vi "Drive Reef Align Alternate_wrapper.vi"() -> ()   [LabVIEW 2023]
uses:
  <vilib>/Rock Robotics/WPI/Framework/Command Status Info.ctl
  <vilib>/Rock Robotics/WPI/Framework/Completion Status.ctl
  <vilib>/Rock Robotics/WPI/Framework/Completion Notifier.ctl
  swerve/Type Definitions/Data/Robot Velocities.ctl
  Implementation/Drive Operations.ctl
panel:
  in  "Operation":T1
  out "Command Info Out":T2
  in  "Description":string
  in  "Auto Data":T6
  in  "Robot Velocities":T5
  in  "Command Info In":T2
  in  "Left side":bool
  in  "Angle Align":bool
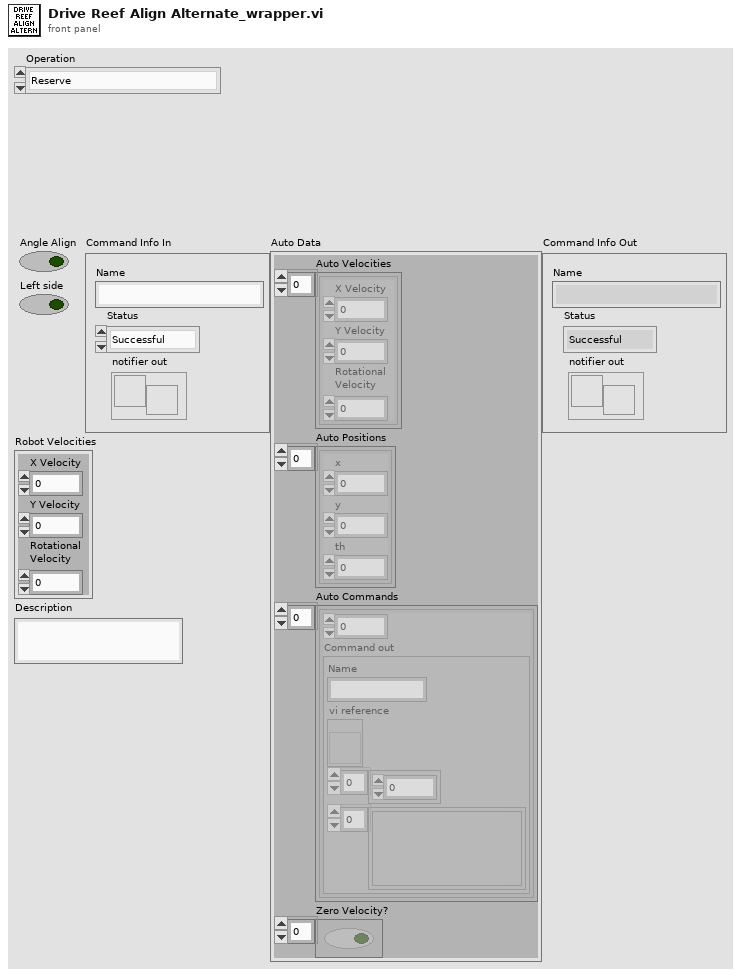
[diagram p1: front panel]
types:
  T1 = typedef "Drive Operations.ctl" = enum16{"Reserve", "Read Current", "Immediate", "Calibrate", "Reef Align", "Auto"}
  T2 = typedef "Command Status Info.ctl" = cluster{"Name":string, "Status":T3, "notifier out":T4}
  T3 = typedef "Completion Status.ctl" = enum16{"Successful", "Aborted", "Incomplete"}
  T4 = typedef "Completion Notifier.ctl" = refnum<notifier>
  T5 = typedef "Robot Velocities.ctl" = cluster{"X Velocity":dbl, "Y Velocity":dbl, "Rotational \nVelocity":dbl}
  T6 = cluster{"Auto Velocities":T5[], "Auto Positions":cluster{"x":dbl, "y":dbl, "th":dbl}[], "Auto Commands":cluster{dbl, "Command out":cluster{"Name":string, "vi reference":refnum<vi>, i32[], variant[]}}[], "Zero Velocity?":bool[]}
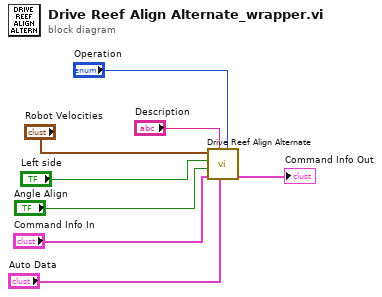
[diagram p0: block diagram]
diagram:
  n1 = call "Drive Reef Align Alternate.vi"("Operation"="Operation", "Auto Data"="Auto Data", "Description"="Description", "Command Info In"="Command Info In", "Angle Align"="Angle Align", "Left side"="Left side", "Robot Velocities"="Robot Velocities") -> ("Command Info Out"=→"Command Info Out":T2)  [unwired: 4 in]
